vi "getOutputVoltage.vi"(8 "error in":errorcluster, 10 "axis in":u8, 11 "connection ID":refnum<k5>) -> (0 "error out":errorcluster, 1 "Voltage (mv)":i64, 2 "axis out":u8, 3 "connection ID":refnum<k5>)   [LabVIEW 2019]
panel:
  in  "Get Command":string="com.attocube.amc.control.getCurrentOutputVoltage"
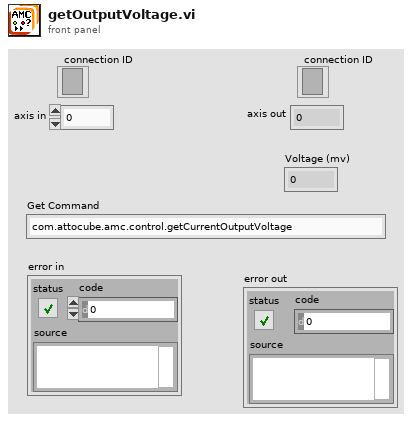
[diagram p1: front panel]
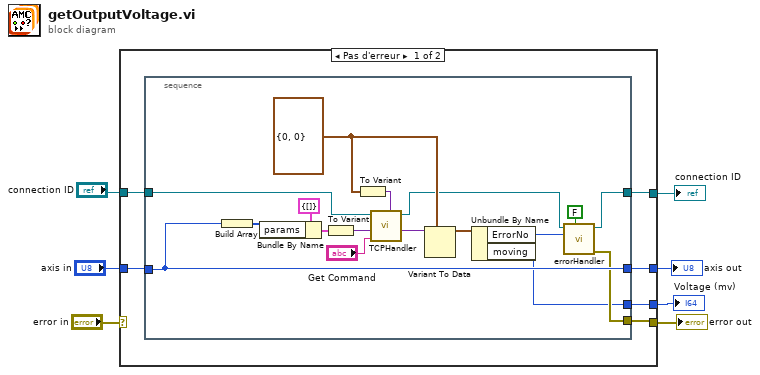
[diagram p0: block diagram]
diagram:
  n1 = case shown="Pas d'erreur" "error in" {
    selector: "error in" -> [_ w32]
    tunnel: "axis in" -> [w13 w33]
    tunnel: [w9 w32] -> w6
    tunnel: [w10 w33] -> w5
    tunnel: [w11 w31] -> w4
    tunnel: "connection ID" -> [w12 w31]
    tunnel: [w8 _] -> w1
    frame No Error {
      n2 = stacked-sequence {
        tunnel: [w15] -> w11
        tunnel: w12 -> [w20]
        tunnel: w13 -> [w22]
        tunnel: [w22] -> w10
        tunnel: [w21] -> w9
        tunnel: [w14] -> w8
        frame #0 {
          w18 = cluster{"ErrorNo":i32, "moving":i64} {"ErrorNo"=0, "moving"=0} ("input cluster")
          n3 = Build Array(w22) -> (w26:u8[])
          n4 = Bundle By Name(cluster=cluster{"params":i32[]} {"params"=[]} ("input cluster"), "params"=w26) -> (w27:cluster{"params":i32[]})
          n5 = To Variant(anything=w27) -> (Variant=w28:variant)
          n6 = To Variant(anything=w18) -> (Variant=w19:variant)
          n7 = call "TCPHandler.vi"("result Types"=w19, "method"="Get Command", "params"=w28, "connection ID"=w20) -> ("result"=w24:variant, "connection ID"=w16:refnum<k5>)  [unwired: 5 in, 1 out]
          n8 = Variant To Data(type=w18, Variant=w24) -> (data=w29:cluster{"ErrorNo":i32, "moving":i64})  [unwired: 1 in, 1 out]
          n9 = Unbundle By Name(w29) -> ("ErrorNo"=w30:i32, "moving"=w14:i64)
          n10 = call "errorHandler.vi"("show popup"=FALSE, "error number"=w30, "connection ID"=w16) -> ("error out"=w21:errorcluster, "connection ID"=w15:refnum<k5>)  [unwired: 7 in]
        }
      }
    }
    frame Error {
    }
  }
  "error out" <- w6
  "axis out" <- w5
  "connection ID" <- w4
  "Voltage (mv)" <- w1
